vi "Write Config.vi"(8 "error in (no error)":errorcluster, 10 "Config":variant, 11 "JsonReportPlugin in":refnum<class "JsonReportPlugin.lvclass">) -> (0 "error out":errorcluster, 3 "JsonReportPlugin out":refnum<class "JsonReportPlugin.lvclass">)   [LabVIEW 2015, in "JsonReportPlugin.lvclass"]
uses:
  JsonReportPlugin.lvclass
  JsonReportPlugin.lvclass/JsonReportPlugin.ctl
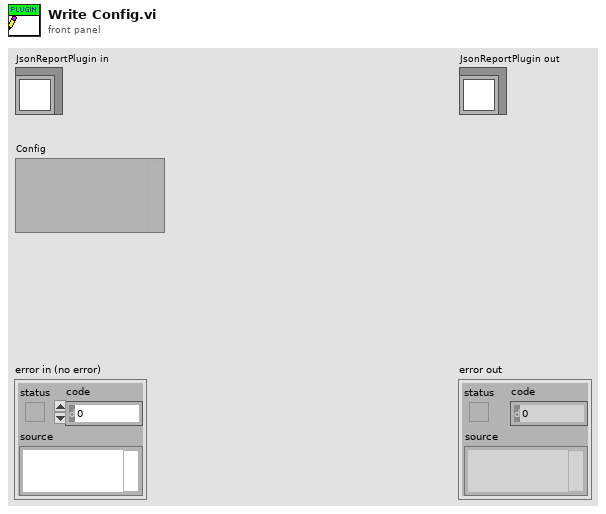
[diagram p1: front panel]
types:
  T1 = cluster{"Enable":bool, "Report Folder":string, "Include SN":bool, "Include Timestamp":bool, "Include Result":bool}
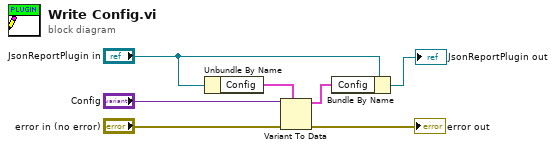
[diagram p0: block diagram]
diagram:
  n1 = Unbundle By Name("JsonReportPlugin in") -> ("Config"=w7:T1)
  n2 = Variant To Data(error in="error in (no error)", type=w7, Variant="Config") -> (data=w3:T1, error out=→"error out":errorcluster)
  n3 = Bundle By Name(cluster="JsonReportPlugin in", "Config"=w3) -> (→"JsonReportPlugin out":refnum<class "JsonReportPlugin.lvclass">)
